vi "Picolog Get Minimum Interval.vi"(8 "Error In":errorcluster, 11 "Instrument Handle In":i16=1) -> (0 "Error Out":errorcluster, 2 "Minimum Interval [s]":dbl format="%.2f", 3 "Instrument Handle Out":i16)   [LabVIEW 2017]
uses:
  usbtc08.dll
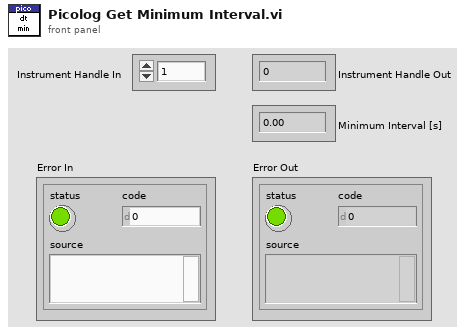
[diagram p1: front panel]
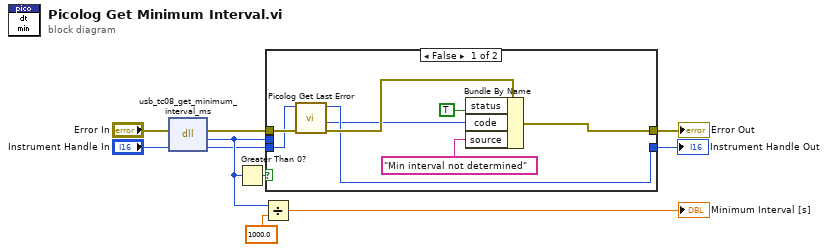
[diagram p0: block diagram]
diagram:
  n1 = dll-call lib="usbtc08.dll" fn="usb_tc08_get_minimum_interval_ms"(error in="Error In", "handle"="Instrument Handle In") -> (error out=w7:errorcluster, "return type"=w4:i32, "handle"=w2:i16)  [unwired: 2 in, 1 out]
  n2 = Greater Than 0?(x=w4) -> (x > 0?=w8:bool)
  n3 = Divide(x=w4, y=1000.0) -> (x/y=→"Minimum Interval [s]":dbl)
  n4 = case shown="False" w8 {
    tunnel: w4 -> [_ _]
    tunnel: w7 -> [w15 w20]
    tunnel: [w18 w20] -> w6
    tunnel: w2 -> [w13 w19]
    tunnel: [w12 w19] -> w1
    frame False {
      n5 = call "Picolog Get Last Error.vi"("Error In"=w15, "Instrument Handle In"=w13) -> ("Error Out"=w14:errorcluster, "Error Code"=w11:i16, "Instrument Handle Out"=w12:i16)  [unwired: 7 in]
      n6 = Bundle By Name(cluster=w14, "status"=TRUE, "code"=w11, "source"="Min interval not determined") -> (w18:errorcluster)
    }
    frame True {
    }
  }
  "Error Out" <- w6
  "Instrument Handle Out" <- w1
